vi "new EnchantedRoom.vi"(8 "error in (no error)":errorcluster, 9 "Spell*":refnum<data-value>, 10 "roomNumber":i32) -> (0 "error out":errorcluster, 3 "EnchantedRoom* out":T1)   [LabVIEW 2016, in "EnchantedRoom.lvclass"]
uses:
  EnchantedRoom.lvclass
  Spell/Spell.lvclass
  EnchantedRoom Reference.ctl
  C:/github/LVOOP-creational-patterns/Maze-Classes/src/Base/Room/Room.lvclass
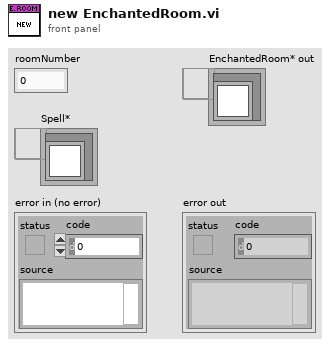
[diagram p1: front panel]
types:
  T1 = typedef "EnchantedRoom.lvclass/EnchantedRoom Reference.ctl" = refnum<data-value>
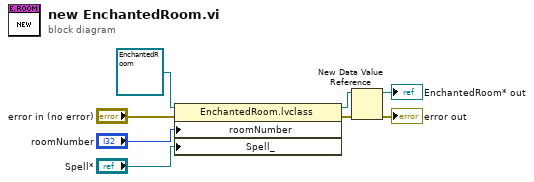
[diagram p0: block diagram]
diagram:
  n1 = property class="EnchantedRoom.lvclass"(reference=refnum<class "EnchantedRoom.lvclass"> refnum ("EnchantedRoom in"), error in="error in (no error)", "roomNumber"="roomNumber", "Spell_"="Spell*") -> (reference out=w4:refnum<class "EnchantedRoom.lvclass">, error out=w3:errorcluster)
  n2 = New Data Value Reference(data value=w4, error in=w3) -> (data value reference=→"EnchantedRoom* out":refnum<data-value>, error out=→"error out":errorcluster)
